vi "Transfer Immediate_wrapper.vi"(0 "Transfer Speed":dbl, 1 "Lower Kicker Speed":dbl) -> (10 "Command Info Out":T1)   [LabVIEW 2025]
uses:
  <vilib>/Rock Robotics/WPI/Framework/Command Status Info.ctl
  <vilib>/Rock Robotics/WPI/Framework/Completion Status.ctl
  <vilib>/Rock Robotics/WPI/Framework/Completion Notifier.ctl
panel:
  in  "Description":string
  in  "Command Info In":T1
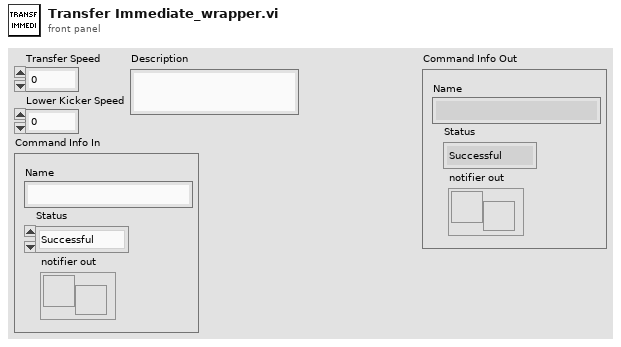
[diagram p1: front panel]
types:
  T1 = typedef "Command Status Info.ctl" = cluster{"Name":string, "Status":T2, "notifier out":T3}
  T2 = typedef "Completion Status.ctl" = enum16{"Successful", "Aborted", "Incomplete"}
  T3 = typedef "Completion Notifier.ctl" = refnum<notifier>
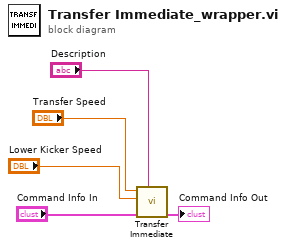
[diagram p0: block diagram]
diagram:
  n1 = call "Transfer Immediate.vi"("Description"="Description", "Command Info In"="Command Info In", "Lower Kicker Speed"="Lower Kicker Speed", "Transfer Speed"="Transfer Speed") -> ("Command Info Out"=→"Command Info Out":T1)  [unwired: 7 in]
